vi "globals.vi"() -> ()   [LabVIEW 2019, in "Useful OAuth VIs.lvlib"]
uses:
  Useful OAuth VIs.lvlib
panel:
  out "Refresh Token":string
  out "Notebook ID":string
  out "AuthToken":string
  out "AuthCode":string
  in  "callback error":errorcluster
  out "Query Strings":map{string, string}(c390)
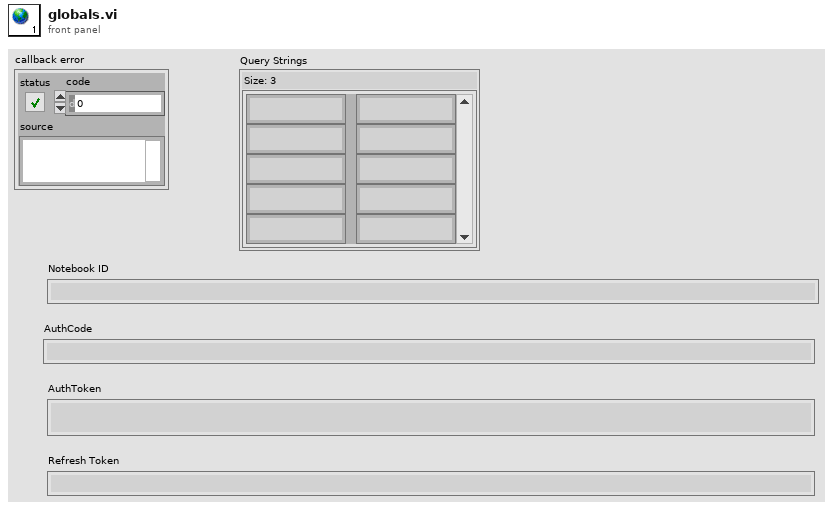
[diagram p1: front panel]
diagram:
